vi "PV MiniTest Valve Test.vi"(7 "Adress of unit":u16=1 min=1 max=999 step=1, 8 "error in (no error)":errorcluster, 10 "Parameter\nread only<->describe":bool, 11 "VISA session":refnum<visa-resource-name>) -> (0 "error out":errorcluster, 2 "response (data)":string, 3 "dup VISA session":refnum<visa-resource-name>)   [LabVIEW 2016, in "Pfeiffer Vacuum.lvlib"]
doc: "This VI allows you to set or check the Valve \"Valve test (Para 609)\" on the MiniTest 300."
uses:
  Pfeiffer Vacuum.lvlib
panel:
  in  "Valve":bool
  # "Valve test"
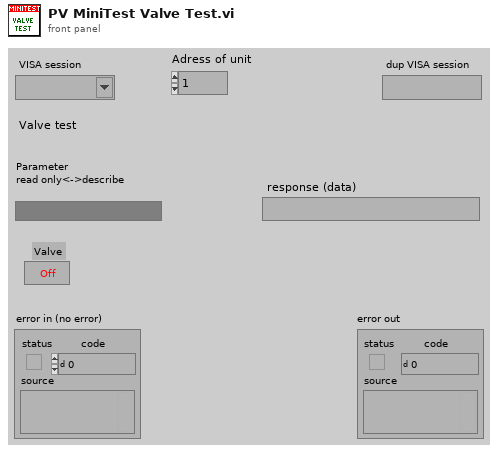
[diagram p1: front panel]
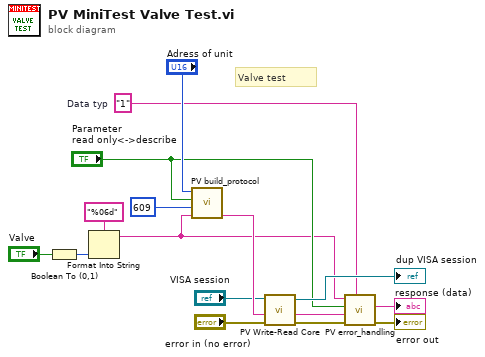
[diagram p0: block diagram]
diagram:
  w10 = "1"  # Data typ
  # "Valve test"
  n1 = Boolean To (0,1)(Boolean="Valve") -> (0, 1=w1:i16)
  n2 = Format Into String(format string="%06d" ("Format-String"), w1) -> (resulting string=w3:string)  [unwired: 2 in, 1 out]
  n3 = call "PV build_protocol.vi"("Data"=w3, "Parameter-number"=u16 609, "parameter\nread<->describe"="Parameter\nread only<->describe", "Adress"="Adress of unit") -> ("output"=w14:string)  [unwired: 3 in]
  n4 = call "PV Write-Read Core.vi"("error in"="error in (no error)", "Write data in"=w14, "VISA session"="VISA session") -> ("error out"=w12:errorcluster, "response (data) out"=w13:string, "dup VISA session"=→"dup VISA session":refnum<visa-resource-name>)  [unwired: 2 in]
  n5 = call "PV error_handling.vi"("Data Typ in"=w10, "error in"=w12, "response (data) in"=w13, "Parameter\nread only<->describe"="Parameter\nread only<->describe", "data in"=w3) -> ("error out"=→"error out":errorcluster, "Data out"=→"response (data)":string)  [unwired: 4 in, 1 out]
